vi "Dashboard Main.vi"() -> ()   [LabVIEW 2013]
uses:
  <vilib>/Rock Robotics/WPI/Camera/WPI_CameraImageSize.ctl
  <vilib>/vision/NI_Vision_Development_Module.lvlib
panel:
  out "Shooter Image":T1(plugin-control)
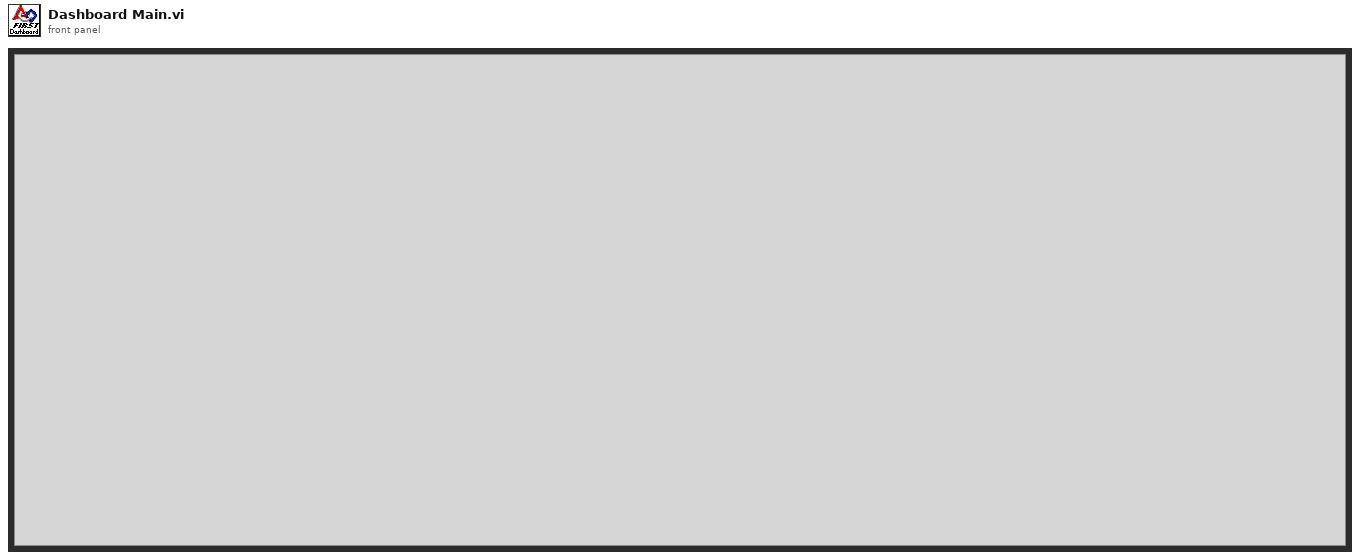
[diagram p1: front panel]
types:
  T1 = typedef "IMAQ Image.ctl" = refnum<image>
  T2 = typedef "Image Type" = u32
  T3 = typedef "WPI_CameraImageSize.ctl" = enum16{"640x480", "320x240", "160x120"}
  T4 = cluster{"fps":i32, "compression":i32, "Image Size":T3}
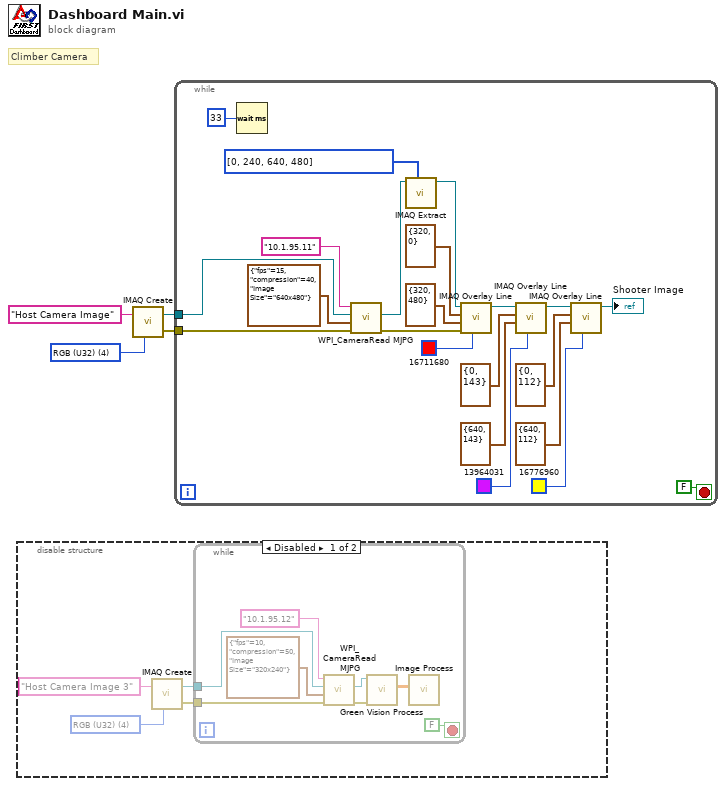
[diagram p0: block diagram]
diagram:
  w3 = T2 4 items=["Grayscale (U8)", "Grayscale (I16)", "Grayscale (SGL)", "Complex (CSG)", "RGB (U32)", "HSL (U32)", "RGB (U64)"] ("Image Type")
  # "Climber Camera"
  n1 = disable-structure shown="Disabled" {
    frame Disabled {
      w7 = T2 4 items=["Grayscale (U8)", "Grayscale (I16)", "Grayscale (SGL)", "Complex (CSG)", "RGB (U32)", "HSL (U32)", "RGB (U64)"] ("Image Type")
      n2 = call "IMAQ Create"("Image Name"="Host Camera Image 3", "Image Type"=w7) -> ("New Image"=w6:T1, "error out"=w5:errorcluster)  [unwired: 2 in, 1 out]
      n3 = while {
        tunnel: w6 -> [w13]
        tunnel: w5 -> [w12]
        stop <- FALSE stop-if-true
        n4 = call <vilib>:"WPI_CameraRead MJPG.vi"("error in"=w12, "Camera Settings"=T4 {"fps"=10, "compression"=50, "Image Size"=enum."320x240"}, "Image"=w13, "address"="10.1.95.12") -> ("error out"=w9:errorcluster, "Image Out"=w10:T1)  [unwired: 5 in, 1 out]
        n5 = call "Green Vision Process.vi"("error in"=w9, "Image In"=w10) -> ("Particle Measurements (Pixels)"=w11:dbl[][])  [unwired: 7 in, 2 out]
        n6 = call "Image Process.vi"("Particle Measurements (Pixels)"=w11) -> ()  [unwired: 6 in, 2 out]
      }
    }
    frame Enabled {
    }
  }
  n7 = call "IMAQ Create"("Image Name"="Host Camera Image", "Image Type"=w3) -> ("New Image"=w2:T1, "error out"=w1:errorcluster)  [unwired: 2 in, 1 out]
  n8 = while {
    tunnel: w2 -> [w30]
    tunnel: w1 -> [w29]
    stop <- FALSE stop-if-true
    n9 = Wait (ms)(milliseconds to wait=u32 33) -> ()  [unwired: 1 out]
    n10 = call <vilib>:"WPI_CameraRead MJPG.vi"("error in"=w29, "Camera Settings"=T4 {"fps"=15, "compression"=40, "Image Size"=enum."640x480"}, "Image"=w30, "address"="10.1.95.11") -> ("error out"=w33:errorcluster, "Image Out"=w19:T1)  [unwired: 5 in, 1 out]
    n11 = call "IMAQ Extract"("Optional Rectangle"=i32[] [0, 240, 640, 480], "Image Src"=w19) -> ("Image Dst Out"=w18:T1)  [unwired: 8 in, 1 out]
    n12 = call "IMAQ Overlay Line"("Color"=u32 16711680, "error in (no error)"=w33, "End Point"=cluster{"X":i32, "Y":i32} {"X"=320, "Y"=480}, "Start Point"=cluster{"X":i32, "Y":i32} {"X"=320, "Y"=0}, "Image"=w18) -> ("Image Out"=w26:T1)  [unwired: 5 in, 1 out]
    n13 = call "IMAQ Overlay Line"("Color"=u32 13964031, "End Point"=cluster{"X":i32, "Y":i32} {"X"=640, "Y"=143} ("Start Point"), "Start Point"=cluster{"X":i32, "Y":i32} {"X"=0, "Y"=143}, "Image"=w26) -> ("Image Out"=w24:T1)  [unwired: 6 in, 1 out]
    n14 = call "IMAQ Overlay Line"("Color"=u32 16776960, "End Point"=cluster{"X":i32, "Y":i32} {"X"=640, "Y"=112} ("Start Point"), "Start Point"=cluster{"X":i32, "Y":i32} {"X"=0, "Y"=112}, "Image"=w24) -> ("Image Out"=→"Shooter Image":T1)  [unwired: 6 in, 1 out]
  }
